vi "ti2_getXPos.vi"(8 "error in (no error)":errorcluster) -> (0 "error out":errorcluster, 3 "x Position (um)":dbl)   [LabVIEW 2023, in "ti2lv.lvlib"]
uses:
  ti2lv.lvlib
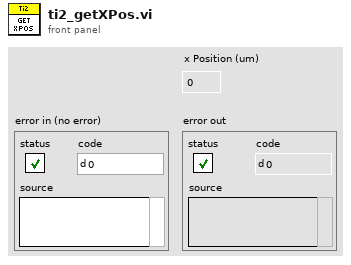
[diagram p1: front panel]
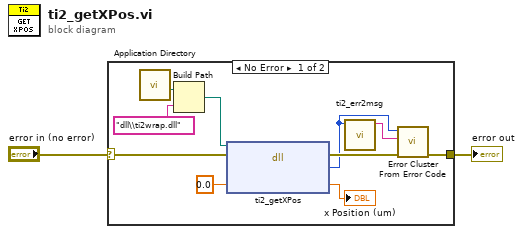
[diagram p0: block diagram]
diagram:
  n1 = case shown="No Error" "error in (no error)" {
    selector: "error in (no error)" -> [w11 w13]
    tunnel: [w12 w13] -> w1
    frame No Error {
      n2 = call <vilib>:"Application Directory.vi"() -> ("Application Directory"=w4:path)
      n3 = Build Path(base path=w4, name or relative path="dll\\ti2wrap.dll") -> (appended path=w3:path)
      n4 = dll-call lib="?" fn="ti2_getXPos"(path in=w3, error in=w11, "xPos_um"=0.0 ("filterPos")) -> (error out=w10:errorcluster, "return type"=w9:i32, "xPos_um"=→"x Position (um)":dbl)  [unwired: 1 in, 1 out]
      n5 = call "ti2_err2msg.vi"("Error Code"=w9) -> ("Error Message"=w8:string)  [unwired: 10 in]
      n6 = call <vilib>:"Error Cluster From Error Code.vi"("error in (no error)"=w10, "error message (\"\")"=w8, "error code (0)"=w9) -> ("error out"=w12:errorcluster)  [unwired: 6 in]
    }
    frame Error {
    }
  }
  "error out" <- w1
